vi "Normalize.vi"(2 "Analog Stick":cluster{"X":dbl, "Y":dbl}, 3 "Past Analog Stick":cluster{"X":dbl, "Y":dbl}[](array[cluster]), 4 "Analog Stick Max":cluster{"X":dbl, "Y":dbl}) -> (0 "Normalized Analog Stick Out":cluster{"X":dbl, "Y":dbl}, 1 "Analog Stick Max Out":cluster{"X":dbl, "Y":dbl})   [LabVIEW 2012]
doc: "Normalize the XY values based on the past max values\nIt also use a running averager from a array of pas values to smooth out data."
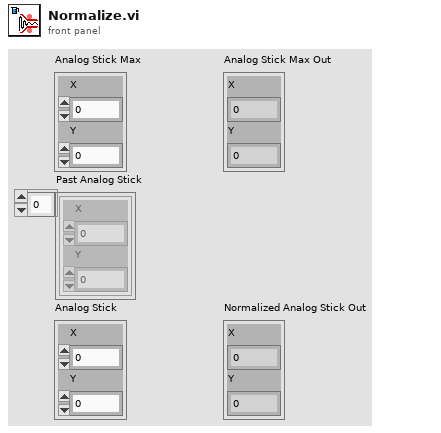
[diagram p1: front panel]
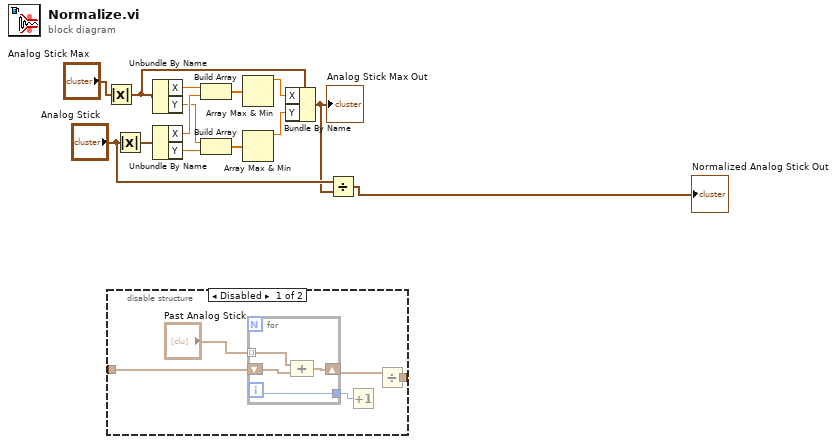
[diagram p0: block diagram]
diagram:
  n1 = Absolute Value(x="Analog Stick Max") -> (abs(x)=w3:cluster{"X":dbl, "Y":dbl})
  n2 = disable-structure shown="Disabled" {
    disable-tunnel: _ -> [w18 _]
    disable-tunnel: [w16 _] -> _
    frame Disabled {
      n3 = for {
        tunnel: "Past Analog Stick" -> [w23] mode=indexing
        shift-right: [w22] -> w17
        shift-left: w18 -> [w21]
        tunnel: [w20] -> w15
        i -> [w20]
        n4 = Compound Arithmetic op=ADD(w23, w21) -> (w22:cluster{"X":dbl, "Y":dbl})
      }
      n5 = Increment(x=w15) -> ()  [unwired: 1 out]
      n6 = Divide(x=w17) -> (x/y=w16:cluster{"X":dbl, "Y":dbl})  [unwired: 1 in]
    }
    frame Enabled {
    }
  }
  n7 = Absolute Value(x="Analog Stick") -> (abs(x)=w14:cluster{"X":dbl, "Y":dbl})
  n8 = Unbundle By Name(w3) -> ("X"=w13:dbl, "Y"=w11:dbl)
  n9 = Unbundle By Name(w14) -> ("X"=w12:dbl, "Y"=w10:dbl)
  n10 = Build Array(w13, w12) -> (w9:dbl[])
  n11 = Build Array(w11, w10) -> (w8:dbl[])
  n12 = Array Max & Min(array=w9) -> (max value=w7:dbl)  [unwired: 3 out]
  n13 = Array Max & Min(array=w8) -> (max value=w6:dbl)  [unwired: 3 out]
  n14 = Bundle By Name(cluster=w3, "X"=w7, "Y"=w6) -> (w4:cluster{"X":dbl, "Y":dbl})
  "Analog Stick Max Out" <- w4
  n15 = Divide(x="Analog Stick", y=w4) -> (x/y=→"Normalized Analog Stick Out":cluster{"X":dbl, "Y":dbl})
